vi "MW100 Communication.vi"(8 "error in (no error)":errorcluster, 11 "Message Queues out":T3) -> (0 "error out":errorcluster)   [LabVIEW 2023]
uses:
  Message Queue/All Message Queues.ctl
  Message Queue/Message Cluster.ctl
  Hybrid Water Heater/Type Definitions/HEWH MW100 Data Cluster.ctl
  Hybrid Water Heater/Custom Instrument Control/MW100/Type Definitions/HEWH Module 4 Relay Status.ctl
  <vilib>/NI/Modbus Library/API/Wrapper/Create TCP Master.vi
  Message Queue/Enqueue Message (Single).vi
  <vilib>/NI/Modbus Library/API/Master/Modbus Master.lvclass
  Message Queue/Message Queue.lvlib
  <vilib>/NI/Modbus Library/API/Wrapper/API Main.lvlib
panel:
  out "MW Output":T1
  in  "Debug":bool
  out "Debug":string[](array[string])
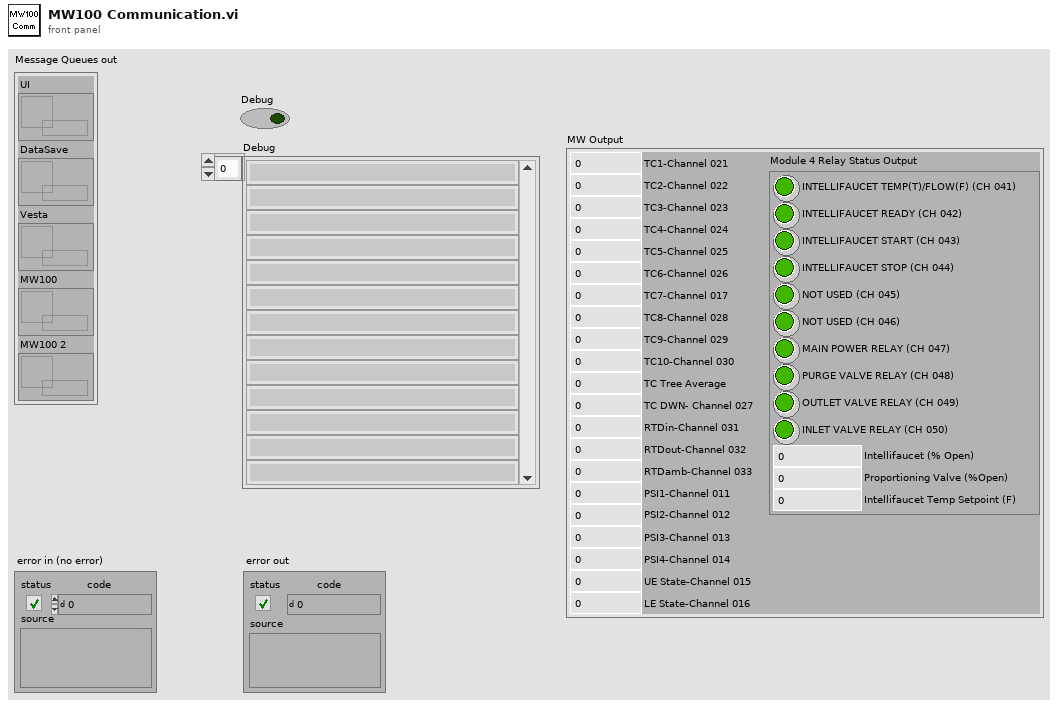
[diagram p1: front panel]
types:
  T1 = typedef "HEWH MW100 Data Cluster.ctl" = cluster{"TC1-Channel 021":dbl, "TC2-Channel 022":dbl, "TC3-Channel 023":dbl, "TC4-Channel 024":dbl, "TC5-Channel 025":dbl, "TC6-Channel 026":dbl, "TC7-Channel 017":dbl, "TC8-Channel 028":dbl, "TC9-Channel 029":dbl, "TC10-Channel 030":dbl, "TC Tree Average":dbl, "TC DWN- Channel 027":dbl, "RTDin-Channel 031":dbl, "RTDout-Channel 032":dbl, "RTDamb-Channel 033":dbl, "PSI1-Channel 011":dbl, "PSI2-Channel 012":dbl, "PSI3-Channel 013":dbl, "PSI4-Channel 014":dbl, "UE State-Channel 015":dbl, "LE State-Channel 016":dbl, "Module 4 Relay Status Output":T2}
  T2 = typedef "HEWH Module 4 Relay Status.ctl" = cluster{"INTELLIFAUCET TEMP(T)/FLOW(F) (CH 041)":bool, "INTELLIFAUCET READY (CH 042)":bool, "INTELLIFAUCET START (CH 043)":bool, "INTELLIFAUCET STOP (CH 044)":bool, "MAIN POWER RELAY (CH 047)":bool, "NOT USED (CH 045)":bool, "NOT USED (CH 046)":bool, "PURGE VALVE RELAY (CH 048)":bool, "OUTLET VALVE RELAY (CH 049)":bool, "INLET VALVE RELAY (CH 050)":bool, "Intellifaucet (% Open)":dbl, "Proportioning Valve (%Open)":dbl, "Intellifaucet Temp Setpoint (F)":dbl}
  T3 = typedef "Message Queue.lvlib/All Message Queues.ctl" = cluster{"UI":refnum<queue>, "DataSave":refnum<queue>, "Vesta":refnum<queue>, "MW100":refnum<queue>, "MW100 2":refnum<queue>}
  T4 = enum8{"Affirmative", "Single Negative", "Multiple Negative", "ASCII", "BINARY", "END"}
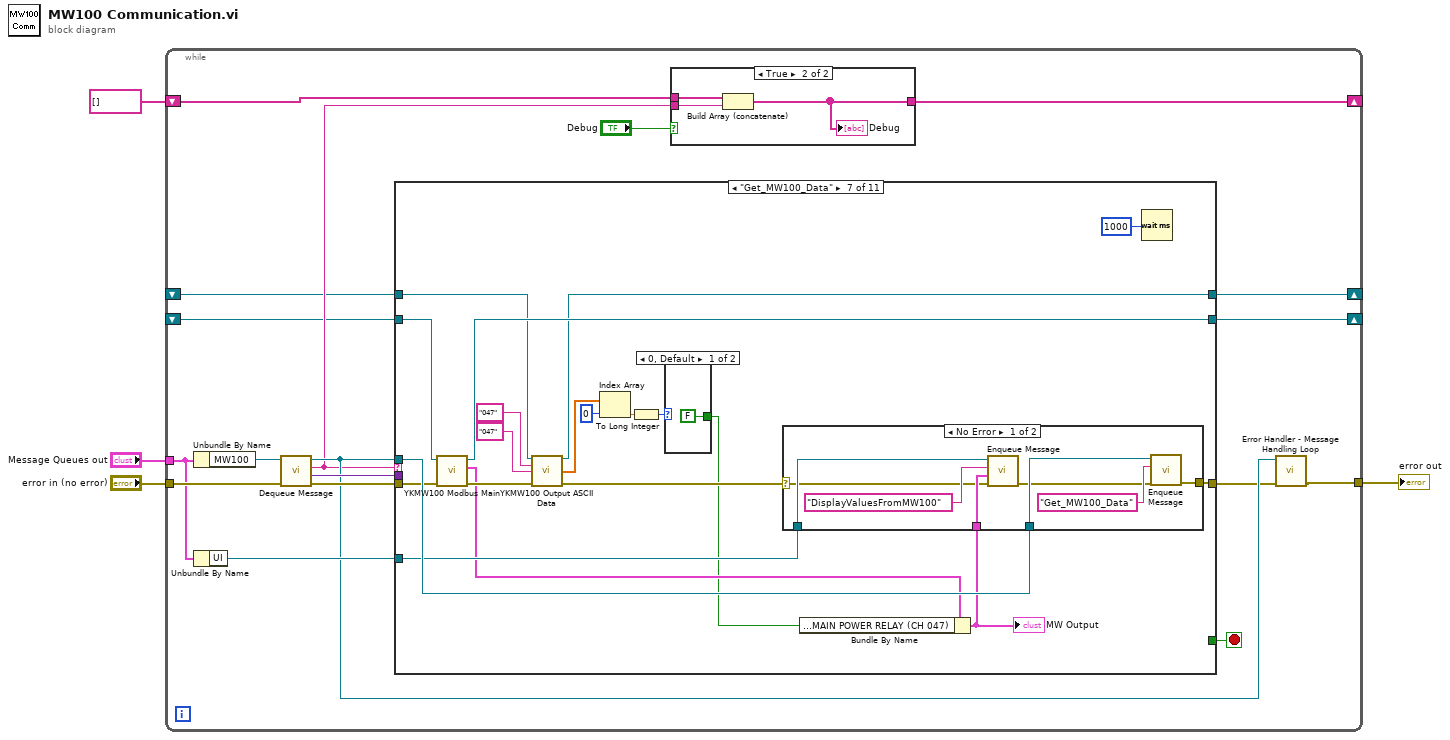
[diagram p0: block diagram]
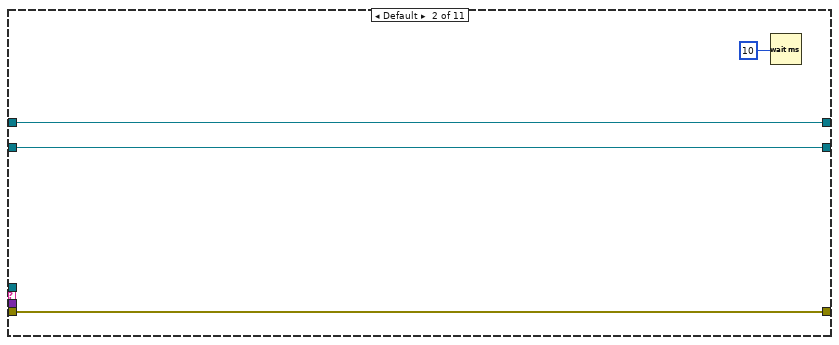
[diagram p4: hidden frame]
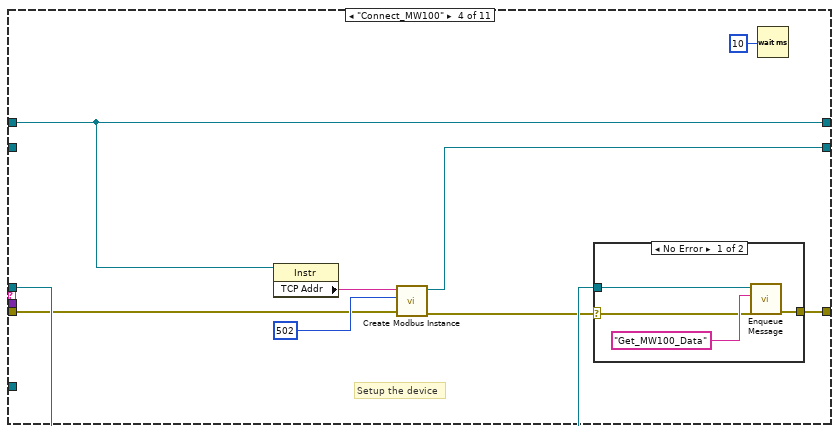
[diagram p6: hidden frame]
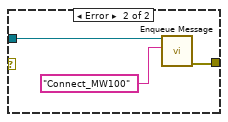
[diagram p7: hidden frame]
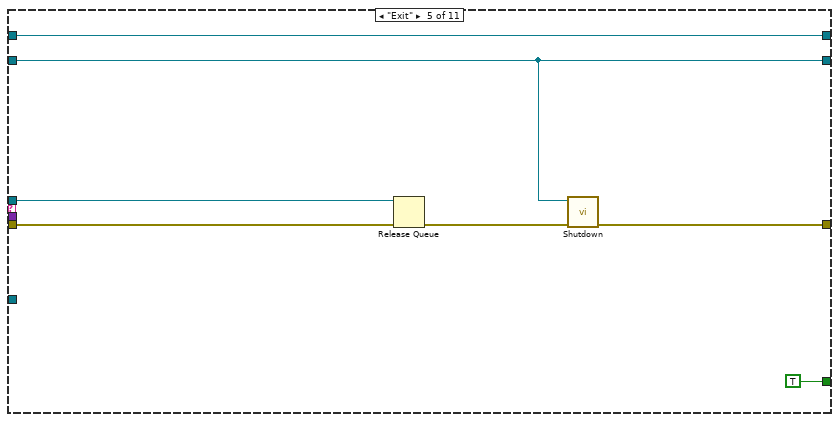
[diagram p8: hidden frame]
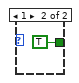
[diagram p10: hidden frame]
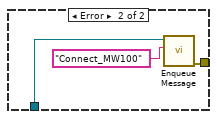
[diagram p11: hidden frame]
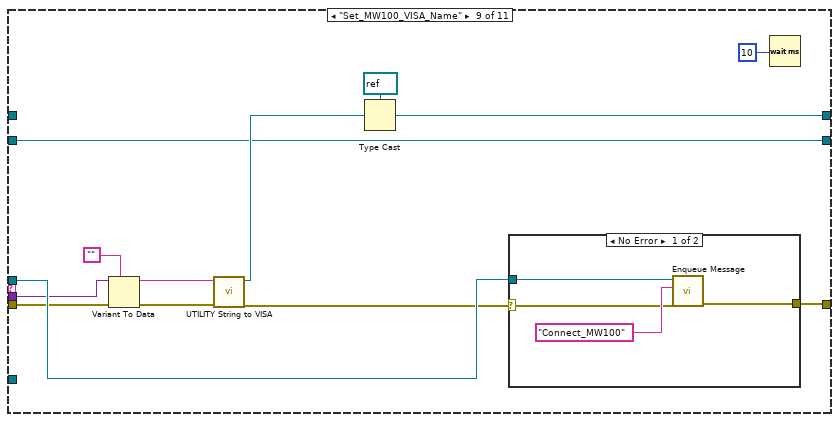
[diagram p13: hidden frame]
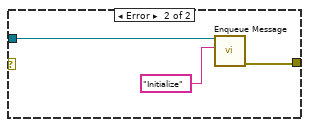
[diagram p14: hidden frame]
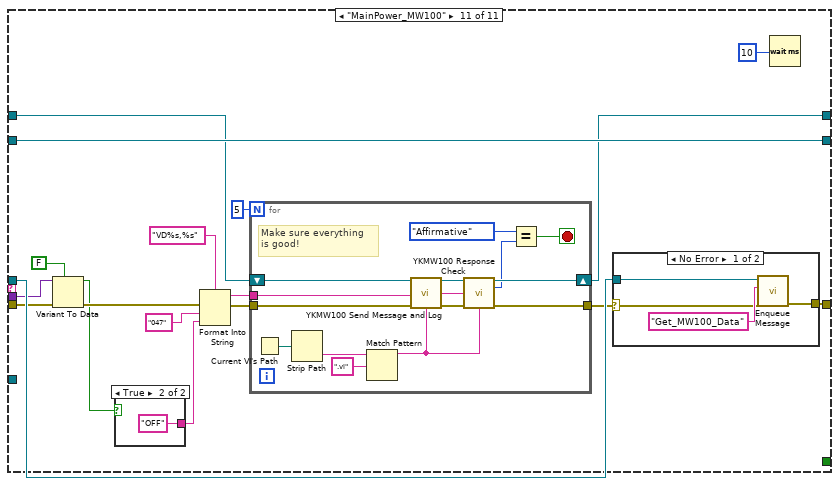
[diagram p16: hidden frame]
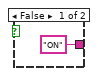
[diagram p17: hidden frame]
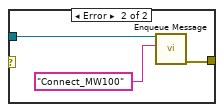
[diagram p18: hidden frame]
diagram:
  n1 = while {
    tunnel: "Message Queues out" -> [w15]
    tunnel: "error in (no error)" -> [w19]
    tunnel: [w11] -> w1
    shift-right: [w16] -> _
    shift-left: string[] [] -> [w17]
    shift-right: [w8] -> _
    shift-left: _ -> [w7]
    shift-right: [w6] -> _
    shift-left: _ -> [w5]
    stop <- w9 stop-if-true
    n2 = Unbundle By Name(w15) -> ("MW100"=w22:refnum<queue>)
    n3 = Unbundle By Name(w15) -> ("UI"=w14:refnum<queue>)
    n4 = call "Dequeue Message.vi"("error in (no error)"=w19, "Message Queue"=w22) -> ("error out"=w20:errorcluster, "Message Data"=w21:variant, "Message"=w10:string, "dup Message Queue"=w13:refnum<queue>)  [unwired: 6 in]
    n5 = case shown="\"Get_MW100_Data\"" w10 {
      tunnel: w13 -> [_ _ _ w44 w58 _ w81 _ w110 _ w138]
      tunnel: w21 -> [_ _ _ _ _ _ _ _ w107 _ w135]
      tunnel: w20 -> [w29 w33 w35 w40 w59 w62 w78 w98 w108 w120 w136]
      tunnel: w14 -> [_ _ _ _ _ _ w80 _ _ _ _]
      tunnel: [w29 w33 w35 w45 w54 w62 w82 w98 w111 w120 w139] -> w12
      tunnel: [_ _ _ _ TRUE _ _ _ _ _ _] -> w9
      tunnel: [w28 w32 w36 w39 w56 w61 w70 w97 w100 w119 w122] -> w8
      tunnel: w7 -> [w28 w32 w36 w39 w56 w61 w73 w97 _ w119 w130]
      tunnel: [w27 w31 w34 w37 w53 w60 w76 w96 w99 w121 w134] -> w6
      tunnel: w5 -> [w27 w31 w34 _ w53 w60 w77 w96 w99 w121 w134]
      frame "---------- Setup ----------" {
      }
      frame Default {
        n6 = Wait (ms)(milliseconds to wait=u32 10) -> ()  [unwired: 1 out]
      }
      frame "Initialize" {
      }
      frame "Connect_MW100" {
        # "Setup the device"
        n7 = property class="Instr"(reference=w39) -> ("TCP Addr"=w42:string)  [unwired: 1 in, 2 out]
        n8 = call-poly <vilib>:"Create Modbus Instance.vi"("error in"=w40, "port (502)"=u16 502, "address"=w42) -> ("error out"=w38:errorcluster, "TCP master instance"=w37:refnum<class "Modbus Master.lvclass">)  [unwired: 7 in]
        n9 = case shown="No Error" w38 {
          selector: w38 -> [w46 _]
          tunnel: [w48 w52] -> w45
          tunnel: w44 -> [w47 w50]
          frame No Error {
            n10 = call-poly "Enqueue Message.vi"("error in (no error)"=w46, "Message"="Get_MW100_Data", "Message Queue"=w47) -> ("error out"=w48:errorcluster)  [unwired: 7 in, 1 out]
          }
          frame Error {
            n11 = call-poly "Enqueue Message.vi"("Message"="Connect_MW100", "Message Queue"=w50) -> ("error out"=w52:errorcluster)  [unwired: 8 in, 1 out]
          }
        }
        n12 = Wait (ms)(milliseconds to wait=u32 10) -> ()  [unwired: 1 out]
      }
      frame "Exit" {
        n13 = Release Queue(queue=w58, error in (no error)=w59) -> (error out=w55:errorcluster)  [unwired: 1 in, 2 out]
        n14 = call-dynamic "Shutdown.vi"("error in"=w55, "Modbus master in"=w53) -> ("error out"=w54:errorcluster)  [unwired: 9 in]
      }
      frame "---------- Data Collection ----------" {
      }
      frame "Get_MW100_Data" {
        n15 = call "YKMW100 Modbus Main.vi"("error in (no error)"=w78, "Modbus master in"=w77) -> ("error out"=w72:errorcluster, "MW Output"=w66:T1, "Modbus master out"=w76:refnum<class "Modbus Master.lvclass">)  [unwired: 7 in]
        n16 = call "YKMW100 Output ASCII Data.vi"("VISA session"=w73, "Start Channel (001)"="047", "End Channel (001)"="047", "error in (no error)"=w72) -> ("dup VISA session"=w70:refnum<visa-resource-name>, "Data List"=w69:dbl[], "error out"=w71:errorcluster)  [unwired: 5 in, 4 out]
        n17 = Index Array(array=w69, index=0) -> (element=w67:dbl)
        n18 = To Long Integer(number=w67) -> (32bit integer=w65:i32)
        n19 = case shown="0, Default" w65 {
          tunnel: [FALSE TRUE] -> w64
          frame 0, Default {
          }
          frame 1 {
          }
        }
        n20 = Bundle By Name(cluster=w66, "Module 4 Relay Status Output.MAIN POWER RELAY (CH 047)"=w64) -> (w63:T1)
        "MW Output" <- w63
        n21 = case shown="No Error" w71 {
          selector: w71 -> [w85 _]
          tunnel: [w91 w95] -> w82
          tunnel: w81 -> [w90 w93]
          tunnel: w80 -> [w88 _]
          tunnel: w63 -> [w86 _]
          frame No Error {
            n22 = call-poly "Enqueue Message.vi"("error in (no error)"=w85, "Message Data"=w86, "Message"="DisplayValuesFromMW100", "Message Queue"=w88) -> ("error out"=w89:errorcluster)  [unwired: 6 in, 1 out]
            n23 = call-poly "Enqueue Message.vi"("error in (no error)"=w89, "Message"="Get_MW100_Data", "Message Queue"=w90) -> ("error out"=w91:errorcluster)  [unwired: 7 in, 1 out]
          }
          frame Error {
            n24 = call-poly "Enqueue Message.vi"("Message"="Connect_MW100", "Message Queue"=w93) -> ("error out"=w95:errorcluster)  [unwired: 8 in, 1 out]
          }
        }
        n25 = Wait (ms)(milliseconds to wait=u32 1000) -> ()  [unwired: 1 out]
      }
      frame "---------- Timer Control ----------" {
      }
      frame "Set_MW100_VISA_Name" {
        n26 = Variant To Data(error in=w108, type="", Variant=w107) -> (data=w101:string, error out=w103:errorcluster)
        n27 = call "UTILITY String to VISA.vi"("error in (no error)"=w103, "VISA Name"=w101) -> ("error out"=w102:errorcluster, "VISA resource name out"=w104:refnum<visa-resource-name>)  [unwired: 8 in]
        n28 = Type Cast(type=refnum<visa-resource-name> refnum ("VISA Refnum in"), x=w104) -> (*(type *) &x=w100:refnum<visa-resource-name>)
        n29 = case shown="No Error" w102 {
          selector: w102 -> [w112 _]
          tunnel: [w114 w118] -> w111
          tunnel: w110 -> [w113 w116]
          frame No Error {
            n30 = call-poly "Enqueue Message.vi"("error in (no error)"=w112, "Message"="Connect_MW100", "Message Queue"=w113) -> ("error out"=w114:errorcluster)  [unwired: 7 in, 1 out]
          }
          frame Error {
            n31 = call-poly "Enqueue Message.vi"("Message"="Initialize", "Message Queue"=w116) -> ("error out"=w118:errorcluster)  [unwired: 8 in, 1 out]
          }
        }
        n32 = Wait (ms)(milliseconds to wait=u32 10) -> ()  [unwired: 1 out]
      }
      frame "---------- Relay Control ----------" {
      }
      frame "MainPower_MW100" {
        n33 = Variant To Data(error in=w136, type=FALSE, Variant=w135) -> (data=w125:bool, error out=w129:errorcluster)
        n34 = case shown="True" w125 {
          tunnel: ["ON" "OFF"] -> w124
          frame False {
          }
          frame True {
          }
        }
        n35 = Format Into String(format string="VD%s,%s", error in=w129, "047", w124) -> (resulting string=w126:string, error out=w128:errorcluster)  [unwired: 1 in]
        n36 = for {
          N: 5 -> [_]
          tunnel: w126 -> [w149]
          shift-right: [w155] -> w122
          shift-left: w130 -> [w156]
          tunnel: w128 -> [w153]
          tunnel: [w154] -> w131
          stop <- w148 stop-if-true
          # "Make sure everything \nis good!"
          n37 = Current VI's Path() -> (path=w144:path)
          n38 = Strip Path(path=w144) -> (name=w145:string)  [unwired: 1 out]
          n39 = Match Pattern(string=w145, regular expression=".vi") -> (before substring=w142:string)  [unwired: 1 in, 3 out]
          n40 = call "YKMW100 Send Message and Log.vi"("VISA session"=w156, "Send Message (\"\")"=w149, "error in (no error)"=w153, "Source (\"\")"=w142) -> ("dup VISA session"=w152:refnum<visa-resource-name>, "Read Buffer"=w150:string, "error out"=w151:errorcluster)  [unwired: 9 in]
          n41 = call "YKMW100 Response Check.vi"("VISA session"=w152, "Message In (\"\")"=w150, "error in (no error)"=w151, "Source (\"\")"=w142) -> ("dup VISA session"=w155:refnum<visa-resource-name>, "Response Type"=w147:T4, "error out"=w154:errorcluster)  [unwired: 7 in, 2 out]
          n42 = Equal?(x=T4."Affirmative", y=w147) -> (x = y?=w148:bool)
        }
        n43 = case shown="No Error" w131 {
          selector: w131 -> [w157 _]
          tunnel: [w159 w163] -> w139
          tunnel: w138 -> [w158 w161]
          frame No Error {
            n44 = call-poly "Enqueue Message.vi"("error in (no error)"=w157, "Message"="Get_MW100_Data", "Message Queue"=w158) -> ("error out"=w159:errorcluster)  [unwired: 7 in, 1 out]
          }
          frame Error {
            n45 = call-poly "Enqueue Message.vi"("Message"="Connect_MW100", "Message Queue"=w161) -> ("error out"=w163:errorcluster)  [unwired: 8 in, 1 out]
          }
        }
        n46 = Wait (ms)(milliseconds to wait=u32 10) -> ()  [unwired: 1 out]
      }
    }
    n47 = case shown="True" "Debug" {
      tunnel: w10 -> [_ w26]
      tunnel: w17 -> [w23 w25]
      tunnel: [w23 w24] -> w16
      frame False {
      }
      frame True {
        n48 = Build Array (concatenate)(w25, w26) -> (w24:string[])
        "Debug" <- w24
      }
    }
    n49 = call "Error Handler - Message Handling Loop.vi"("error in (no error)"=w12, "Message Queue"=w13) -> ("dup error in"=w11:errorcluster)  [unwired: 8 in, 1 out]
  }
  "error out" <- w1
